vi "Valve Type.vi"(11 "PulsedValve in":refnum<class "PulsedValve.lvclass">) -> (2 "Valve Type":string)   [LabVIEW 2020, in "VolatusControl.lvlib" / "PulsedValve.lvclass"]
uses:
  PulsedValve.lvclass
  PulsedValve.lvclass/PulsedValve.ctl
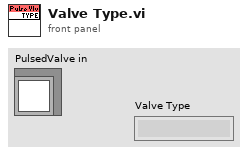
[diagram p1: front panel]
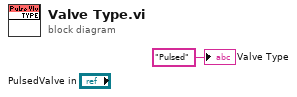
[diagram p0: block diagram]
diagram:
  "Valve Type" <- "Pulsed" ("Valve Type")
